vi "FarFiledCamColse.vi"   [LabVIEW 2018]
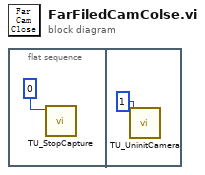
[diagram p0: block diagram]
diagram:
  n1 = flat-sequence {
    frame #0 {
      n2 = call "TU_StopCapture.vi"("CameraIndex"=0) -> ()  [unwired: 8 in, 2 out]
    }
    frame #1 {
      n3 = call "TU_UninitCamera.vi"("nCamCount"=1) -> ()  [unwired: 8 in, 2 out]
    }
  }
